vi "Store Configuration Parameters.vi"(8 "error in (no error)":errorcluster, 10 "refnum":T1, 11 "CCD Configuration in":refnum<class "CCD Configuration.lvclass">) -> (0 "error out":errorcluster, 2 "refnum out":T1, 3 "CCD Configuration out":refnum<class "CCD Configuration.lvclass">)   [LabVIEW 2016, in "CCD.lvlib" / "CCD Configuration.lvclass"]
uses:
  <userlib>/Common Components/Hardware/CCD/CCD Configuration.lvclass
  <vilib>/Utility/config.llb/Config Data RefNum.ctl
  <userlib>/Common Components/Hardware/CCD/CCD Configuration.lvclass/CCD Configuration.ctl
  <userlib>/Common Components/Hardware/Abstract Hardware/Hardware.lvclass/Hardware.ctl
  <userlib>/Common Components/Hardware/CCD/CCD/CCD.lvclass/CCD.ctl
  <userlib>/Common Components/Hardware/DevInfo/DevInfo.lvclass/DevInfo.ctl
  <userlib>/Common Components/Hardware/CCD/CCD Configuration/Read Hardware.lvlib_CCD.lvlib_CCD.lvclass.vi
  <userlib>/Common Components/Hardware/Abstract Hardware/Read Label.vi
  <userlib>/Common Components/Hardware/Abstract Hardware/Read DevInfo.vi
  <userlib>/Common Components/Hardware/DevInfo/Read HW Type.vi
  <userlib>/Common Components/Hardware/DevInfo/Read Device Name.vi
  <userlib>/Common Components/Hardware/DevInfo/Read COMM Address.vi
  <userlib>/Common Components/Hardware/DevInfo/Read Sub-COMM Address.vi
  <userlib>/Common Components/Hardware/CCD/CCD/CCD.lvclass
  C:/Program Files (x86)/National Instruments/LabVIEW 2016/user.lib/Common Components/Hardware/Abstract Hardware/Hardware.lvclass
  <userlib>/Common Components/Hardware/DevInfo/DevInfo.lvclass
  <vilib>/Utility/config.llb/NI_LVConfig.lvlib
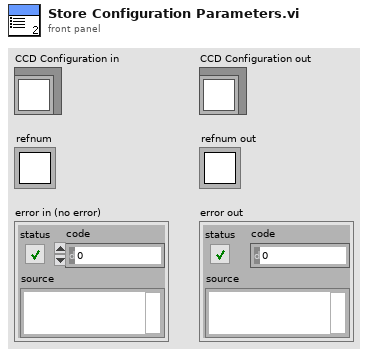
[diagram p1: front panel]
types:
  T1 = typedef "NI_LVConfig.lvlib/Config Data RefNum.ctl" = refnum<k1>
  T2 = typedef "CCD.lvlib/CCD.lvclass/camer data.ctl" = cluster{"VideoMode":u16, "gain":u32, "gamma":sgl, "Contrast":dbl, "Exposure":u32, "Saturation":u32}
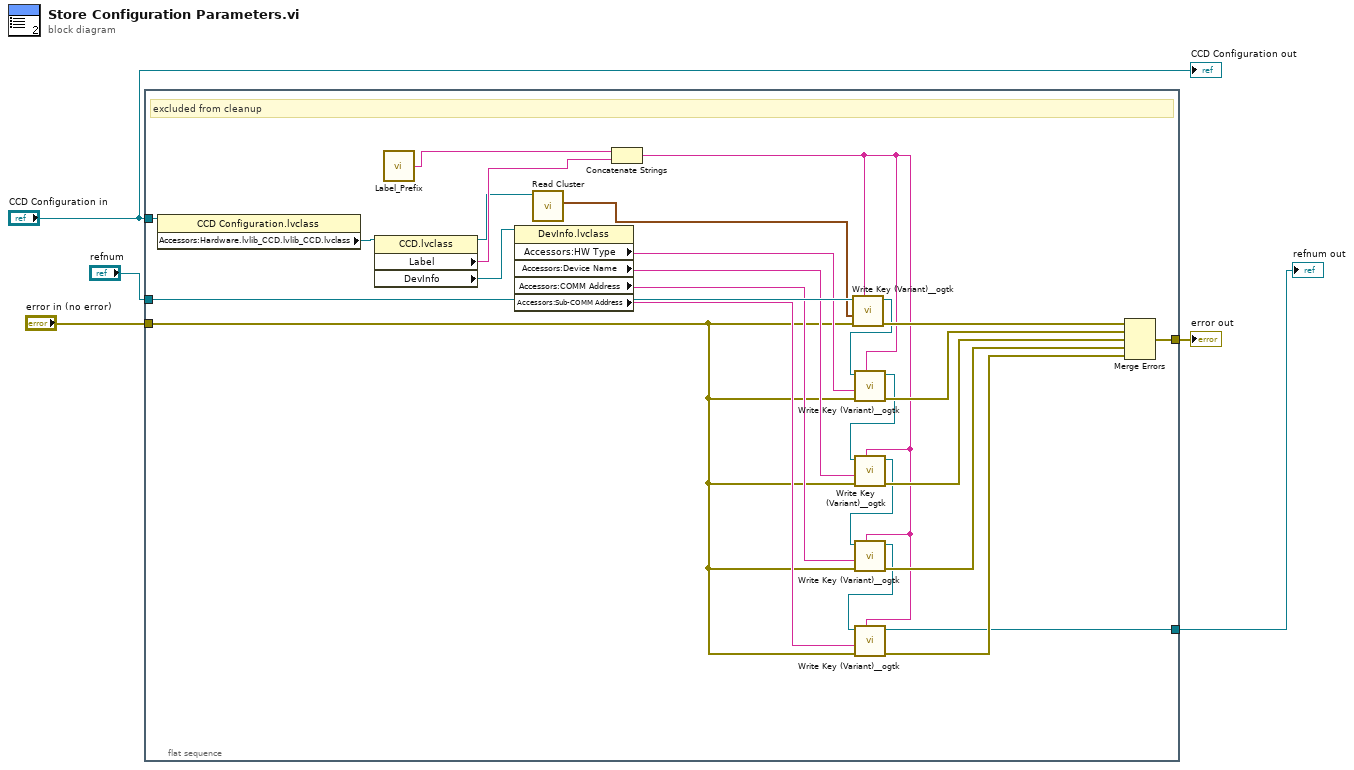
[diagram p0: block diagram]
diagram:
  n1 = flat-sequence {
    tunnel: "refnum" -> [w30]
    tunnel: "error in (no error)" -> [w10]
    tunnel: "CCD Configuration in" -> [w29]
    tunnel: [w28] -> w5
    tunnel: [w6] -> w1
    frame #0 {
      # "excluded from cleanup"
      n2 = property class="CCD Configuration.lvclass"(reference=w29) -> ("Accessors:Hardware.lvlib_CCD.lvlib_CCD.lvclass"=w12:refnum<class "CCD.lvclass">)  [unwired: 1 in, 2 out]
      n3 = property class="CCD.lvclass"(reference=w12) -> (reference out=w9:refnum<class "CCD.lvclass">, "Label"=w18:string, "DevInfo"=w17:refnum<class "DevInfo.lvclass">)  [unwired: 1 in, 1 out]
      n4 = call <userlib>:"Label_Prefix.vi"() -> ("Label Prefix String"=w7:string)
      n5 = property class="DevInfo.lvclass"(reference=w17) -> ("Accessors:HW Type"=w16:string, "Accessors:Device Name"=w15:string, "Accessors:COMM Address"=w14:string, "Accessors:Sub-COMM Address"=w13:string)  [unwired: 1 in, 2 out]
      n6 = call <userlib>:"Read Cluster.vi"("CCD in"=w9) -> ("Cluster"=w8:T2)  [unwired: 8 in, 2 out]
      n7 = Concatenate Strings(w7, w18) -> (w11:string)
      n8 = call <userlib>:"Write Key (Variant)__ogtk.vi"("section"=w11, "error in (no error)"=w10, "key-value"=w8, "refnum"=w30) -> ("error out"=w27:errorcluster, "refnum out"=w22:T1)  [unwired: 6 in]
      n9 = call <userlib>:"Write Key (Variant)__ogtk.vi"("section"=w11, "error in (no error)"=w10, "key-value"=w16, "refnum"=w22) -> ("error out"=w26:errorcluster, "refnum out"=w21:T1)  [unwired: 6 in]
      n10 = call <userlib>:"Write Key (Variant)__ogtk.vi"("section"=w11, "error in (no error)"=w10, "key-value"=w15, "refnum"=w21) -> ("error out"=w25:errorcluster, "refnum out"=w20:T1)  [unwired: 6 in]
      n11 = call <userlib>:"Write Key (Variant)__ogtk.vi"("section"=w11, "error in (no error)"=w10, "key-value"=w14, "refnum"=w20) -> ("error out"=w24:errorcluster, "refnum out"=w19:T1)  [unwired: 6 in]
      n12 = call <userlib>:"Write Key (Variant)__ogtk.vi"("section"=w11, "error in (no error)"=w10, "key-value"=w13, "refnum"=w19) -> ("error out"=w23:errorcluster, "refnum out"=w6:T1)  [unwired: 6 in]
      n13 = Merge Errors(w27, w26, w25, w24, w23) -> (w28:errorcluster)
    }
  }
  "CCD Configuration out" <- "CCD Configuration in"
  "error out" <- w5
  "refnum out" <- w1
